vi "Set-options.vi"(8 "error in (no error)":errorcluster, 10 "Options":T1, 11 "Object ref in":T2) -> (0 "error out":errorcluster, 3 "Object ref out":T2)   [LabVIEW 2013, in "PowderDeposition.lvlib" / "PD-Main.lvclass"]
uses:
  PD-Main.lvclass
  Object-reference.ctl
  Options.ctl
  PD-Main.lvclass/PD-Main.ctl
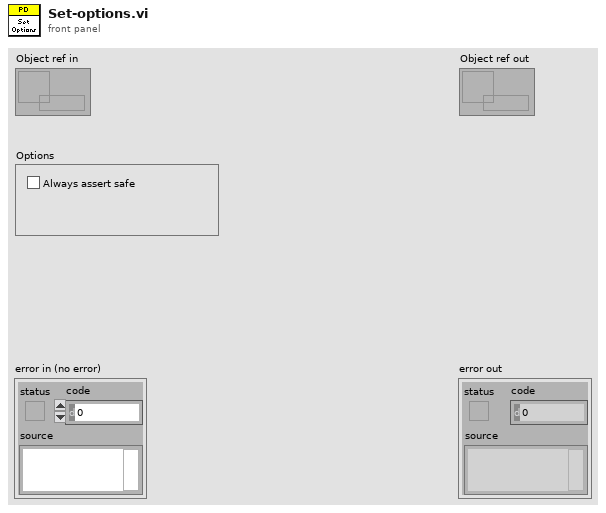
[diagram p1: front panel]
types:
  T1 = typedef "PowderDeposition.lvlib/PD-Main.lvclass/Options.ctl" = cluster{"Assert safe":bool}
  T2 = typedef "PowderDeposition.lvlib/PD-Main.lvclass/Object-reference.ctl" = refnum<data-value>
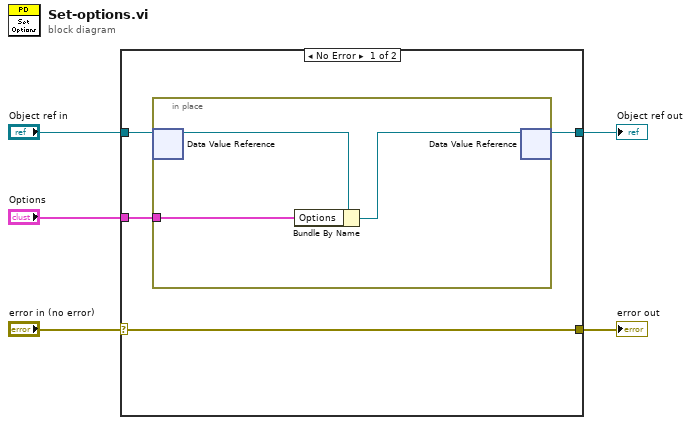
[diagram p0: block diagram]
diagram:
  n1 = case shown="No Error" "error in (no error)" {
    selector: "error in (no error)" -> [w6 w14]
    tunnel: [w6 w14] -> w4
    tunnel: [w7 w13] -> w2
    tunnel: "Object ref in" -> [w9 w13]
    tunnel: "Options" -> [w8 _]
    frame No Error {
      n2 = in-place {
        in-place-border: w8 -> [w11]
        n3 = in-place-dvr #1(w9) -> (w12:refnum<class "PD-Main.lvclass">)  [unwired: 1 out]
        n4 = Bundle By Name(cluster=w12, "Options"=w11) -> (w10:refnum<class "PD-Main.lvclass">)
        n5 = in-place-dvr #1(w10) -> (w7:T2)  [unwired: 1 out]
      }
    }
    frame Error {
    }
  }
  "error out" <- w4
  "Object ref out" <- w2
